vi "Broadcast Response.vi"(8 "error in (no error)":errorcluster, 9 "Acquired Result.lvclass":refnum<class "Acquired Result.lvclass">, 10 "Topic":string, 11 "Log Record in":refnum<class "Log Record.lvclass">) -> (0 "error out":errorcluster, 3 "Log Record out":refnum<class "Log Record.lvclass">)   [LabVIEW 2020, in "Log Record.lvclass"]
uses:
  Log Record.lvclass
  Log Record.lvclass/Log Record.ctl
  NHMFL_Core/Libraries/Instruments/Results/Acquired Result/Acquired Result.lvclass
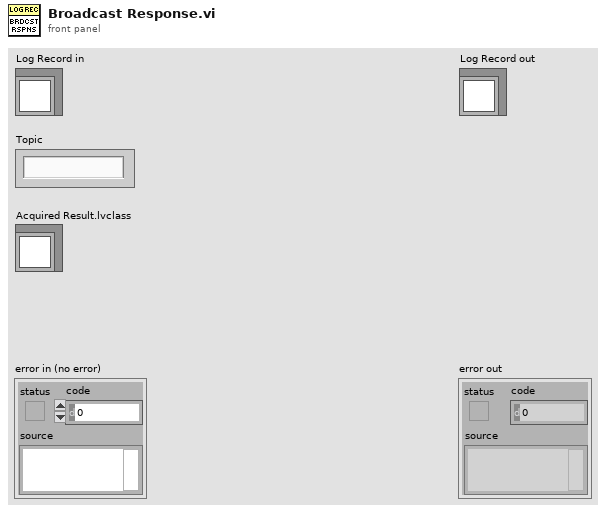
[diagram p1: front panel]
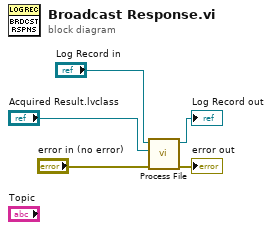
[diagram p0: block diagram]
diagram:
  n1 = call-dynamic "Process File.vi"("error in (no error)"="error in (no error)", "Result in"="Acquired Result.lvclass", "Log Record in"="Log Record in") -> ("error out"=→"error out":errorcluster, "Log Record out"=→"Log Record out":refnum<class "Log Record.lvclass">)  [unwired: 6 in, 1 out]
